vi "maxenergy.vi"(9 "数组":cdb[](array[numeric]), 11 "parameters":T1 {"簇"."pulse shaping filter" items=["none", "Raised Cosine", "Root Raised Cos", "Gsussian"]; "簇"."modulation type" items=["FSK", "PSK", "QAM", "MSK", "PAM", "ASK"]}) -> (3 "output":cdb[](array[numeric]))   [LabVIEW 2014]
uses:
  <vilib>/Analysis/2dsp.llb/Decimate (single shot, CDB).vi
  <vilib>/Analysis/NI_AALPro.lvlib
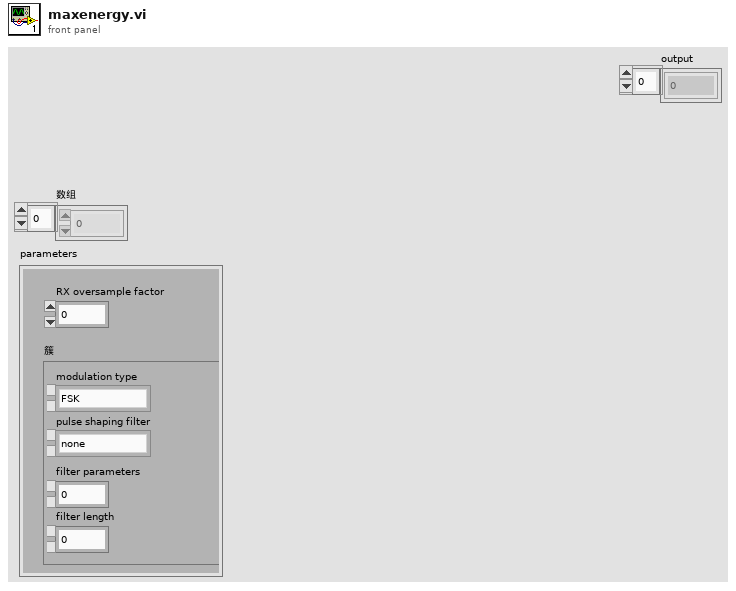
[diagram p1: front panel]
types:
  T1 = cluster{"RX oversample factor":i32, "簇":cluster{"modulation type":u16, "pulse shaping filter":u16, "filter parameters":dbl, "filter length":i32}}
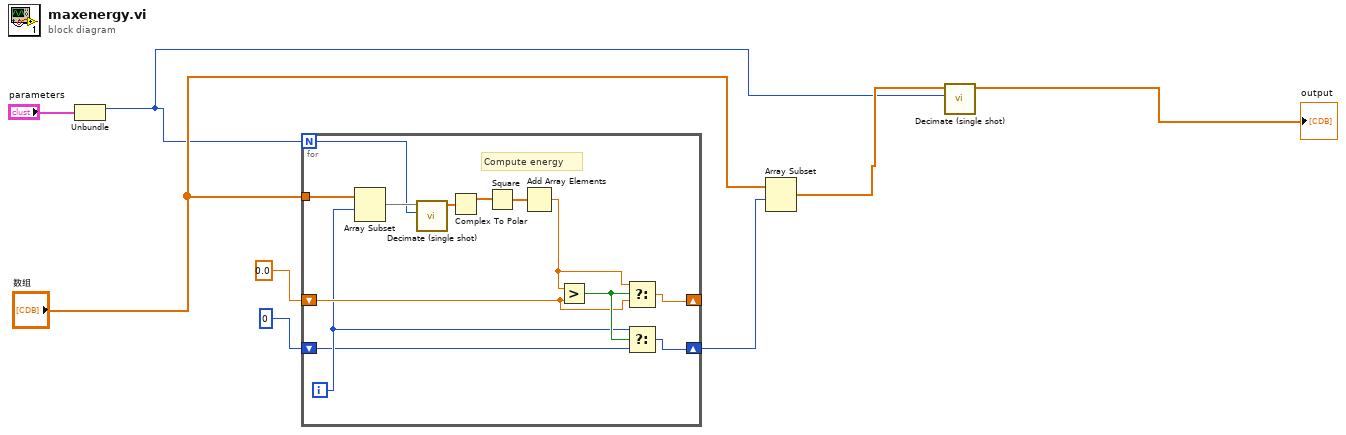
[diagram p0: block diagram]
diagram:
  n1 = Unbundle("parameters") -> ("RX oversample factor"=w1:i32)  [unwired: 1 out]
  n2 = for {
    N: w1 -> [w9]
    tunnel: "数组" -> [w21]
    shift-right: [w15] -> w4
    shift-left: 0 -> [w16]
    shift-right: [w14] -> _
    shift-left: 0.0 -> [w19]
    i -> [w17]
    # "Compute energy"
    n3 = Array Subset(array=w21, index=w17) -> (w13:cdb[])  [unwired: 1 in]
    n4 = call-poly <vilib>:"Decimate (single shot).vi"("decimating factor"=w9, "X"=w13) -> ("Decimated Array"=w12:cdb[])  [unwired: 8 in, 1 out]
    n5 = Complex To Polar(r * e^(i*theta)=w12) -> (r=w11:dbl[])  [unwired: 1 out]
    n6 = Square(x=w11) -> (x^2=w10:dbl[])
    n7 = Add Array Elements(numeric array=w10) -> (sum=w18:dbl)
    n8 = Greater?(x=w18, y=w19) -> (0:w20:bool)
    n9 = Select(t=w18, s=w20, f=w19) -> (s? t:f=w14:dbl)
    n10 = Select(t=w17, s=w20, f=w16) -> (s? t:f=w15:i32)
  }
  n11 = Array Subset(array="数组", index=w4) -> (w2:cdb[])  [unwired: 1 in]
  n12 = call-poly <vilib>:"Decimate (single shot).vi"("decimating factor"=w1, "X"=w2) -> ("Decimated Array"=→"output":cdb[])  [unwired: 8 in, 1 out]
